vi "Pyramid Initial Command.vi"(6 "y offset":dbl, 7 "z offset":dbl, 9 "x offset":dbl, 10 "reference_corners":dbl[][](array[numeric]), 11 "increment initial":dbl) -> (3 "3D Comet 2":refnum<class "3D Plot Datatype.lvclass">[](xcontrol))   [LabVIEW 2017]
uses:
  <vilib>/Math Plots/3D Math Plots/3D Comet/3D Comet XCtrl/3D Comet.xctl
  Globals.vi
  <vilib>/Math Plots/3D Math Plots/3D Comet/3D Comet Datatype/Public/Plot Helper (Vector).vi
  <vilib>/Math Plots/3D Math Plots/3D Comet/3D Comet Datatype/3D Comet Datatype.lvclass
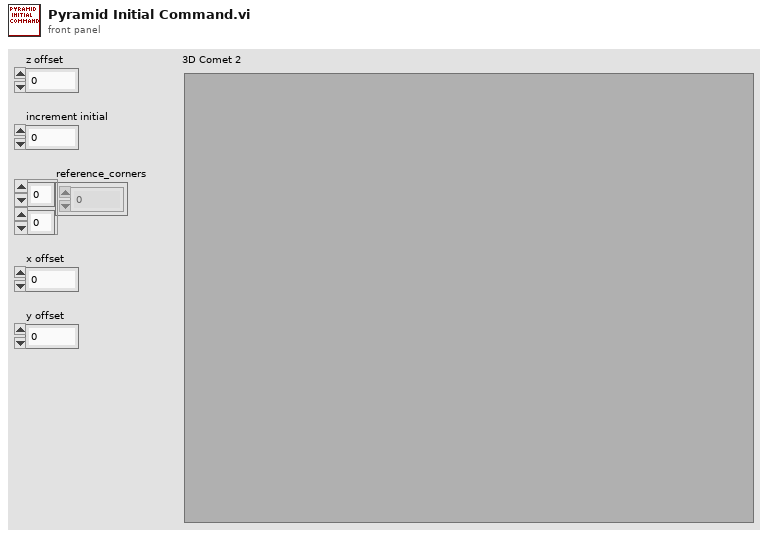
[diagram p1: front panel]
types:
  T1 = cluster{"increment initial":dbl, "vangle initial":dbl, "overlap initial":dbl, "width initial":dbl, "height initial":dbl, "layers initial":dbl}
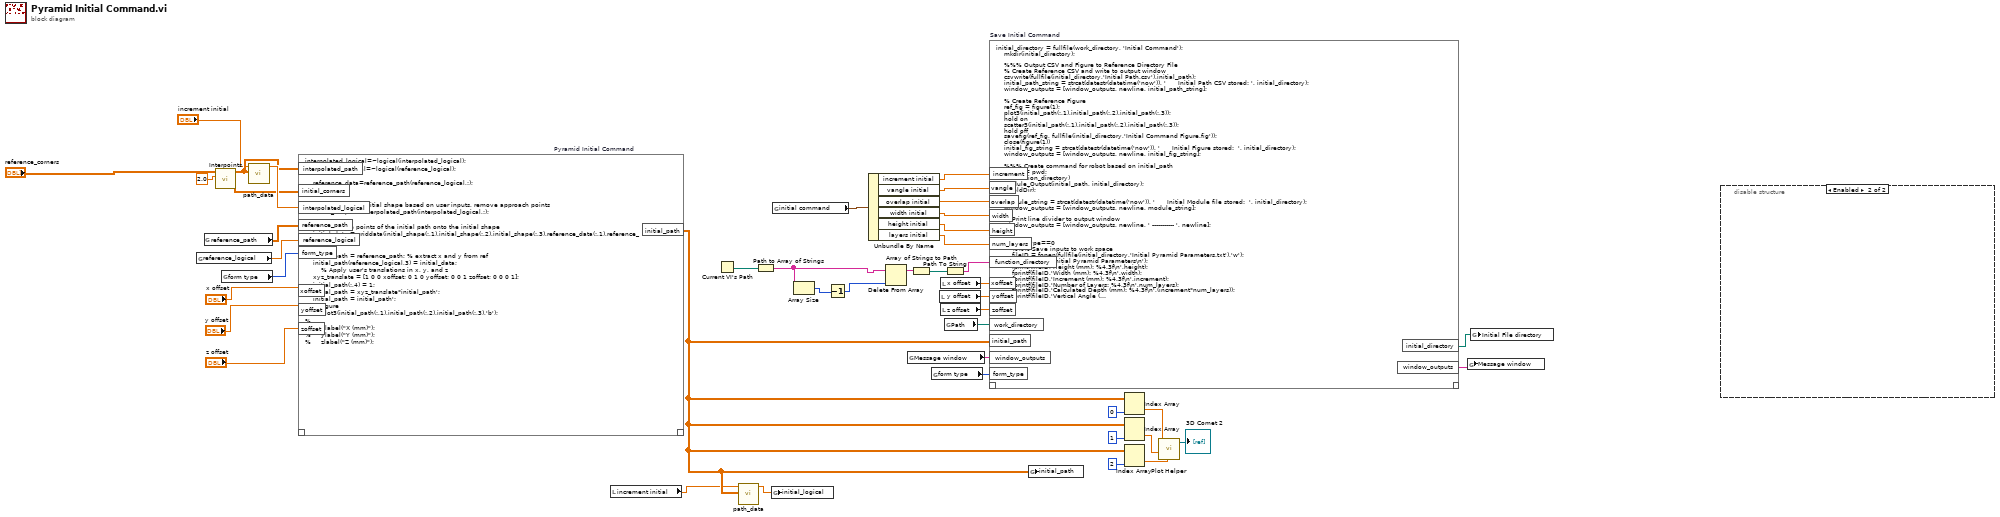
[diagram p0: block diagram]
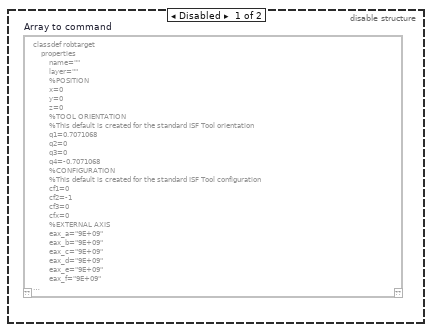
[diagram p2: hidden frame]
diagram:
  n1 = global read "Globals.vi" "reference_logical"() -> (w27:dbl[])
  n2 = global read "Globals.vi" "reference_path"() -> (w28:dbl[][])
  n3 = call "Interpoints.vi"("Min_dist"=2.0, "reference_corners"="reference_corners") -> ("Corners"=w30:dbl[][], "Reference path"=w32:dbl[][])  [unwired: 8 in]
  n4 = global read "Globals.vi" "form type"() -> (w34:u16)
  n5 = call "path_data.vi"("path in"=w32, "increment"="increment initial") -> ("path logical"=w33:dbl[])  [unwired: 9 in]
  n6 = script code="interpolated_logical=~logical(interpolated_logical);\n    reference_logical=~logical(reference_logical);\n   \n    reference_data=reference_path(reference_logical,:);\n\n    \n    %%% Generate initial shape based on user inputs, remove approach points\n    initial_shape = interpolated_path(interpolated_logical,:);\n    \n    % Project the points of the initial path onto the initial shape\n    initial_data = griddata(initial_shape(:,1),initial_shape(:,2),initial_shape(:,3),reference_data(:,1),reference_data(:,2));\n\n    initial_path = reference_path; % extract x and y from ref\n    initial_path(reference_logical,3) = initial_data; \n        % Apply user's translations in x, y, and z\n    xyz_translate = [1 0 0 xoffset; 0 1 0 yoffset; 0 0 1 zoffset; 0 0 0 1];\n    initial_path(:,4) = 1;\n    initial_path = xyz_translate*initial_path';\n    initial_path = initial_path';\n%     figure\n%     plot3(initial_path(:,1),initial_path(:,2),initial_path(:,3),'b');    \n% \n%     xlabel(\"X (mm)\");\n%     ylabel(\"Y (mm)\");\n%     zlabel(\"Z (mm)\");" "Pyramid Initial Command"("initial_corners"=w30, "reference_path"=w28, "reference_logical"=w27, "interpolated_path"=w32, "interpolated_logical"=w33, "form_type"=w34, "xoffset"="x offset", "yoffset"="y offset", "zoffset"="z offset") -> ("initial_path"=w3:dbl[][])  [unwired: 1 in, 1 out]
  n7 = local read "increment initial"() -> (w2:dbl)
  n8 = Current VI's Path() -> (path=w15:path)
  n9 = call "path_data.vi"("path in"=w3, "increment"=w2) -> ("path logical"=w1:dbl[])  [unwired: 9 in]
  n10 = Path to Array of Strings(0:w15) -> (2:w14:string[])  [unwired: 1 out]
  n11 = global write "Globals.vi" "initial_logical"(w1) -> ()
  n12 = global read "Globals.vi" "initial command"() -> (w25:T1)
  n13 = Array Size(array=w14) -> (size(s)=w12:i32)
  n14 = Decrement(x=w12) -> (x-1=w11:i32)
  n15 = Unbundle By Name(w25) -> ("increment initial"=w24:dbl, "vangle initial"=w23:dbl, "overlap initial"=w22:dbl, "width initial"=w21:dbl, "height initial"=w20:dbl, "layers initial"=w19:dbl)
  n16 = Delete From Array(array=w14, index=w11) -> (array with subset deleted=w13:string[])  [unwired: 1 in, 1 out]
  n17 = global read "Globals.vi" "Message window"() -> (w36:string)
  n18 = Array of Strings to Path(0:w13) -> (2:w10:path)  [unwired: 1 in]
  n19 = global read "Globals.vi" "form type"() -> (w26:u16)
  n20 = local read "y offset"() -> (w17:dbl)
  n21 = local read "x offset"() -> (w18:dbl)
  n22 = local read "z offset"() -> (w16:dbl)
  n23 = global read "Globals.vi" "Path"() -> (w35:path)
  n24 = Path To String(path=w10) -> (string=w9:string)
  n25 = script code="initial_directory = fullfile(work_directory, 'Initial Command');\n    mkdir(initial_directory);\n\n    %%% Output CSV and Figure to Reference Directory File\n    % Create Reference CSV and write to output window\n    csvwrite(fullfile(initial_directory,'Initial Path.csv'),initial_path);\n    initial_path_string = strcat(datestr(datetime('now')), '      Initial Path CSV stored: ', initial_directory);\n    window_outputs = [window_outputs, newline, initial_path_string];   \n\n    % Create Reference Figure    \n    ref_fig = figure(1);\n    plot3(initial_path(:,1),initial_path(:,2),initial_path(:,3));\n    hold on\n    scatter3(initial_path(:,1),initial_path(:,2),initial_path(:,3));\n    hold off\n    savefig(ref_fig, fullfile(initial_directory,'Initial Command Figure.fig'));\n    close(figure(1))\n    initial_fig_string = strcat(datestr(datetime('now')), '      Initial Figure stored:  ', initial_directory);\n    window_outputs = [window_outputs, newline, initial_fig_string];\n    \n    %%% Create command for robot based on initial_path\n    oldDir = pwd;\n    cd(function_directory)\n    Module_Output(initial_path, initial_directory);\n    cd(oldDir);\n\n    module_string = strcat(datestr(datetime('now')), '      Initial Module file stored:  ', initial_directory);\n    window_outputs = [window_outputs, newline, module_string];\n\n    % Print line divider to output window\n    window_outputs = [window_outputs, newline, ' ----------- ', newline];\n    \n\n    if form_type==0\n        %%% Save inputs to work space\n        fileID = fopen(fullfile(initial_directory,'Initial Pyramid Parameters.txt'),'w');\n        fprintf(fileID,'Initial Pyramid Parameters\\n');\n        fprintf(fileID,'Height (mm): %4.3f\\n',height);\n        fprintf(fileID,'Width (mm): %4.3f\\n',width);\n        fprintf(fileID,'Increment (mm): %4.3f\\n',increment);\n        fprintf(fileID,'Number of Layers: %4.3f\\n',num_layers);\n        fprintf(fileID,'Calculated Depth (mm): %4.3f\\n',(increment*num_layers));\n        fprintf(fileID,'Vertical Angle (degrees): %4.3f\\n',vangle);\n        fprintf(fileID,'Overlap (mm): %4.3f\\n',overlap);\n        fprintf(fileID,'X offset (mm): %4.3f\\n',xoffset);\n        fprintf(fileID,'Y offset (mm): %4.3f\\n',yoffset);\n        fprintf(fileID,'Z offset (mm): %4.3f\\n',zoffset);\n        fclose(fileID);\n    end" "Save Initial Command"("work_directory"=w35, "initial_path"=w3, "window_outputs"=w36, "form_type"=w26, "xoffset"=w18, "yoffset"=w17, "zoffset"=w16, "increment"=w24, "vangle"=w23, "overlap"=w22, "width"=w21, "height"=w20, "num_layers"=w19, "function_directory"=w9) -> ("initial_directory"=w8:path, "window_outputs"=w37:string)  [unwired: 1 in, 1 out]
  n26 = global write "Globals.vi" "initial_path"(w3) -> ()
  n27 = Index Array(array=w3, index (col)=0 ("disabled index (col)")) -> (element=w44:dbl[])  [unwired: 1 in]
  n28 = Index Array(array=w3, index (col)=1 ("disabled index (col)")) -> (element=w43:dbl[])  [unwired: 1 in]
  n29 = Index Array(array=w3, index (col)=2 ("disabled index (col)")) -> (element=w42:dbl[])  [unwired: 1 in]
  n30 = call-poly <vilib>:"Plot Helper.vi"("z vector"=w42, "y vector"=w43, "x vector"=w44) -> ("3D Plot lvclass Array out"=→"3D Comet 2":refnum<class "3D Plot Datatype.lvclass">[])  [unwired: 3 in, 5 out]
  n31 = global write "Globals.vi" "Message window"(w37) -> ()
  n32 = global write "Globals.vi" "Initial File directory"(w8) -> ()
  n33 = disable-structure shown="Enabled" {
    frame Disabled {
      n34 = script code="classdef robtarget\n    properties\n        name=\"\"\n        layer=\"\"\n        %POSITION\n        x=0\n        y=0\n        z=0\n        %TOOL ORIENTATION\n        %This default is created for the standard ISF Tool orientation\n        q1=0.7071068\n        q2=0\n        q3=0\n        q4=-0.7071068\n        %CONFIGURATION\n        %This default is created for the standard ISF Tool configuration\n        cf1=0\n        cf2=-1\n        cf3=0\n        cfx=0\n        %EXTERNAL AXIS\n        eax_a=\"9E+09\"\n        eax_b=\"9E+09\"\n        eax_c=\"9E+09\"\n        eax_d=\"9E+09\"\n        eax_e=\"9E+09\"\n        eax_f=\"9E+09\"\n        \n        %COMMON MOTION CONTROL\n        speed=42.5;\n        zone=\"fine\";\n        wobj=\"wobj_ISF1\";\n        tool=\"tool_ISF2fs\";\n        \n    end\n    methods\n    end\nend\n\nfly_point = logical(zeros(length(path),1));\n    for i = 2:length(path)-1\n        %%% Locally store next 3 points\n        x1 = round(path(i-1,1),3);\n        y1 = round(path(i-1,2),3);\n        z1 = round(path(i-1,3),3);\n\n        x2 = round(path(i,1),3);\n        y2 = round(path(i,2),3);\n        z2 = round(path(i,3),3);\n\n        x3 = round(path(i+1,1),3);\n        y3 = round(path(i+1,2),3);\n        z3 = round(path(i+1,3),3);\n        \n        u = [ x2-x1 y2-y1 z2-z1 ];\n        v = [ x3-x2 y3-y2 z3-z2 ]; \n        \n        theta(i) = atan2d(norm(cross(u,v)),dot(u,v));\n        \n        if theta(i) < 80\n            fly_point(i,1) = logical(1);\n            \n        end\n        theta = theta';\n\n    end\n    fly_point(end,1) = logical(0);\n    \n    %%% Assign matrix to array of robtargets (command)\n    command = robtarget.empty(length(path),0);\n    for i = 1:length(path)\n        command(i,1).name = ['p',num2str(i)];\n        command(i,1).x = path(i,1);\n        command(i,1).y = path(i,2);\n        command(i,1).z = path(i,3);\n        if fly_point(i)\n            command(i,1).zone = 'z0';\n        end\n    end" "Array to command"() -> ()  [unwired: 1 in, 1 out]
    }
    frame Enabled {
    }
  }
